vi "APS get start point index.vi"(8 "error in (no error)":errorcluster caption="错误输入（无错误）", 10 "Index":i32, 11 "Axis_ID":i32) -> (0 "error out":errorcluster caption="错误输出", 2 "Index out":i32, 3 "function return":i32)   [LabVIEW 2011, in "APS168.lvlib"]
doc: "I32 FNTYPE APS_get_start_point_index( I32 Axis_ID, I32 *Index );"
uses:
  APS168.lvlib
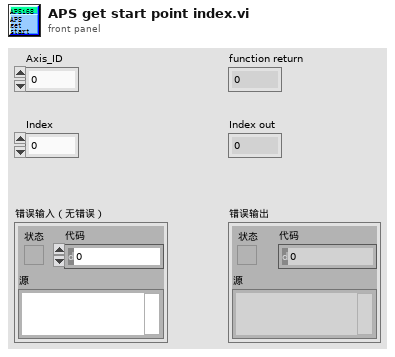
[diagram p1: front panel]
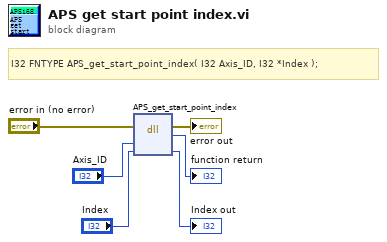
[diagram p0: block diagram]
diagram:
  # "I32 FNTYPE APS_get_start_point_index( I32 Axis_ID, I32 *Index );"
  n1 = dll-call lib="PTH1Labs E软件ADLINK 204CAPS_1_7_1_LIB line 连续运动204APS168.*" fn="APS_get_start_point_index"(error in="error in (no error)", "Axis_ID"="Axis_ID", "Index"="Index") -> (error out=→"error out":errorcluster, →"function return":i32, "Index"=→"Index out":i32)  [unwired: 3 in, 1 out]
